vi "Add Registered Process.vi"(4 "Sync Notifier":refnum<notifier>, 6 "Process Runs (T)":bool=TRUE, 8 "error in (no error)":errorcluster, 9 "Process Name (Optional)":string, 10 "Process VI (Static VI Ref)":refnum<vi>, 11 "SMO":refnum<class "SMO.lvclass">) -> (0 "error out":errorcluster, 3 "SMO out":refnum<class "SMO.lvclass">)   [LabVIEW 2021, in "smo.lvlib" / "SMO.lvclass"]
doc: "---------------------------------------------------------------\nCopyright © 2014 JKI All rights reserved.\nAuthor: Philippe Guerit <philippe.guerit@jki.net>\nThis library is provided \"AS IS\" , WITHOUT WARRANTIES OR \nCONDITIONS OF ANY KIND, either express or implied.\nJKI. -- jki.net"
uses:
  SMO.lvclass
  SMO.lvclass/SMO.ctl
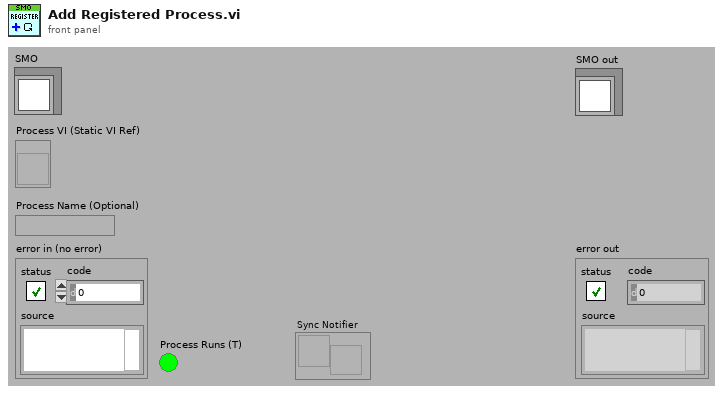
[diagram p1: front panel]
types:
  T1 = typedef "smo.lvlib/SMO.lvclass/PrivateData--Ref.ctl" = refnum<data-value>
  T2 = typedef "smo.lvlib/SMO.lvclass/PrivateData--Cluster.ctl" = cluster{"Parent Call":T3, "Registered Processes":T4[], "Sync Notifier":refnum<notifier>, "Process Error Notifier":refnum<notifier>, "Protected Events":T5, "Public Events":T6, "SMO State":T7, "[Attributes]":variant, "Launcher Close":refnum<notifier>, "Caller Watchdog":refnum<queue>, "Accessibility":T8, "NbStaticDependencies":u32}
  T3 = typedef "smo.lvlib/SMO.lvclass/Parent Call--Enum.ctl" = enum16{"Allows parent to run", "Does not request parent to run"}
  T4 = typedef "smo.lvlib/SMO.lvclass/RegisteredProcessData--Cluster.ctl" = cluster{"Name":string, "Static VI Ref":refnum<vi>, "Running":bool, "NotifierRef":u32}
  T5 = typedef "smo.lvlib/SMO.lvclass/Protected Events.ctl" = cluster{"StopProcesses":refnum<user-event>, "AbortProcesses":refnum<user-event>, "Config Changed":refnum<user-event>, "Dependency":refnum<user-event>}
  T6 = typedef "smo.lvlib/SMO.lvclass/Public Events.ctl" = cluster{"Error":refnum<user-event>, "State":refnum<user-event>, "Reserve State":refnum<user-event>}
  T7 = typedef "smo.lvlib/SMO.lvclass/SMOState --Enum.ctl" = enum16{"unknown", "Created", "Started", "Stopped"}
  T8 = typedef "smo.lvlib/SMO.lvclass/Accessibility--Cluster.ctl" = cluster{"Lock Key":string, "Reserve State":T9}
  T9 = typedef "smo.lvlib/SMO.lvclass/Reserve State--Enum.ctl" = enum16{"Unreserved", "Reserved", "Self-locked"}
  T10 = cluster{"Clone Name":string, "Process VI (Static VI Ref)":refnum<vi>, "Process Runs (T)":bool, u32}
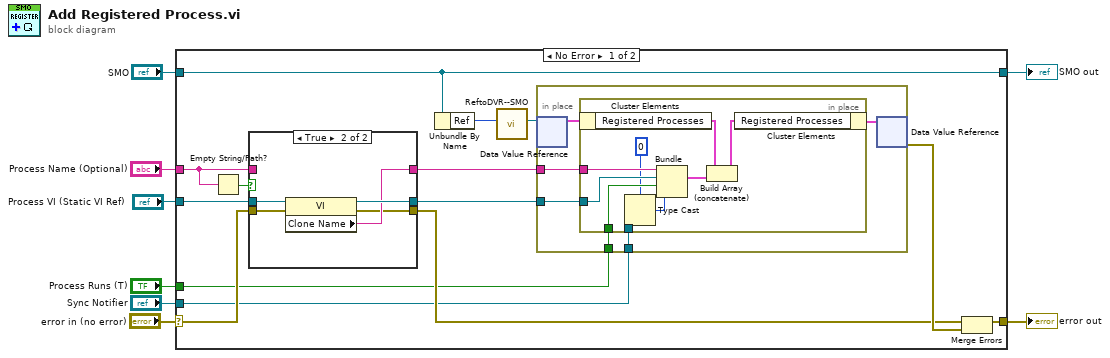
[diagram p0: block diagram]
diagram:
  n1 = case shown="No Error" "error in (no error)" {
    selector: "error in (no error)" -> [w15 w47]
    tunnel: "Process VI (Static VI Ref)" -> [w20 _]
    tunnel: [w21 w47] -> w7
    tunnel: "Process Name (Optional)" -> [w16 _]
    tunnel: [w9 w46] -> w4
    tunnel: "SMO" -> [w9 w46]
    tunnel: "Process Runs (T)" -> [w13 _]
    tunnel: "Sync Notifier" -> [w12 _]
    frame No Error {
      n2 = Empty String/Path?(string/path=w16) -> (empty?=w18:bool)
      n3 = case shown="True" w18 {
        tunnel: w20 -> [w39 w45]
        tunnel: [w39 w44] -> w19
        tunnel: [w40 w43] -> w17
        tunnel: w16 -> [w40 _]
        tunnel: w15 -> [w38 w42]
        tunnel: [w38 w41] -> w14
        frame False {
        }
        frame True {
          n4 = property class="VI"(reference=w45, error in=w42) -> (reference out=w44:refnum<vi>, error out=w41:errorcluster, "Clone Name"=w43:string)
        }
      }
      n5 = Unbundle By Name(w9) -> ("Ref"=w11:u32)
      n6 = call "ReftoDVR--SMO.vi"("Ref"=w11) -> ("Ref"=w10:T1)  [unwired: 10 in]
      n7 = in-place {
        in-place-border: w17 -> [w27]
        in-place-border: w19 -> [w26]
        in-place-border: w13 -> [w24]
        in-place-border: w12 -> [w23]
        n8 = in-place-dvr #1(w10) -> (w28:T2)  [unwired: 1 out]
        n9 = in-place {
          in-place-border: w27 -> [w35]
          in-place-border: w26 -> [w34]
          in-place-border: w24 -> [w32]
          in-place-border: w23 -> [w30]
          n10 = in-place-cluster #2(w28) -> ("Registered Processes"=w37:T4[])
          n11 = Type Cast(type=u32 0, x=w30) -> (*(type *) &x=w29:u32)
          n12 = Bundle("Clone Name"=w35, "Process VI (Static VI Ref)"=w34, "Process Runs (T)"=w32, w29) -> (w33:T10)  [unwired: 1 in]
          n13 = Build Array (concatenate)(w37, w33) -> (w36:T4[])
          n14 = in-place-cluster #2("Registered Processes"=w36) -> (w25:T2)
        }
        n15 = in-place-dvr #1(w25) -> (w22:errorcluster)  [unwired: 1 out]
      }
      n16 = Merge Errors(w14, w22) -> (w21:errorcluster)
    }
    frame Error {
    }
  }
  "error out" <- w7
  "SMO out" <- w4
